vi "RSZVB Set Noise Figure Measurement Mode.vi"(8 "error in (no error)":errorcluster {"code" format="%.0x"}, 9 "Measurement Mode (On)":bool=TRUE, 10 "Channel (1)":i32=1, 11 "VISA session":refnum<visa-resource-name>) -> (0 "error out":errorcluster {"code" format="%.0x"}, 3 "dup VISA session":refnum<visa-resource-name>)   [LabVIEW 2011]
doc: "This VI selects sequential or simultaneous measurement mode. \n\nNote(s):\n\n(1) This VI is available only with option R&S ZVAB-K30.\n\nRemote-control command(s):\n[SENSe<Ch>:]NFIGure:SEQuential ON | OFF"
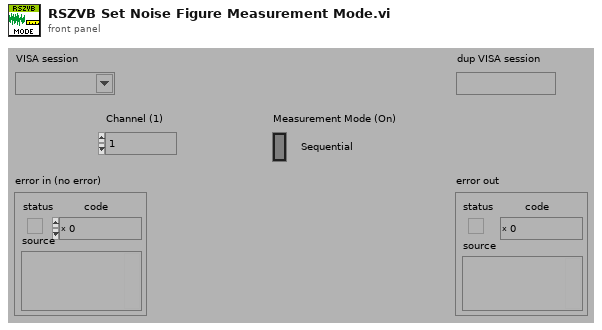
[diagram p1: front panel]
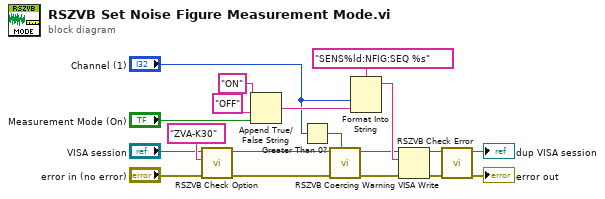
[diagram p0: block diagram]
diagram:
  n1 = call "RSZVB Check Option.vi"("error in (no error)"="error in (no error)", "Options"="ZVA-K30", "VISA session"="VISA session") -> ("error out"=w5:errorcluster, "dup VISA session"=w6:refnum<visa-resource-name>)  [unwired: 7 in]
  n2 = Append True/False String(1:"Measurement Mode (On)", 2:"OFF" ("false string"), 3:"ON" ("true string")) -> (0:w7:string)  [unwired: 1 in]
  n3 = Greater Than 0?(x="Channel (1)") -> (x > 0?=w15:bool)
  n4 = call "RSZVB Coercing Warning.vi"("In Range?"=w15, "error in (no error)"=w5, "VISA session"=w6) -> ("error out"=w14:errorcluster, "dup VISA session"=w13:refnum<visa-resource-name>)  [unwired: 7 in]
  n5 = Format Into String(format string="SENS%ld:NFIG:SEQ %s", "Channel (1)", w7) -> (resulting string=w16:string)  [unwired: 2 in, 1 out]
  n6 = VISA Write(VISA resource name=w13, write buffer=w16, error in (no error)=w14) -> (VISA resource name out=w10:refnum<visa-resource-name>, error out=w11:errorcluster)  [unwired: 1 out]
  n7 = call "RSZVB Check Error.vi"("error in (no error)"=w11, "VISA session"=w10) -> ("error out"=→"error out":errorcluster, "dup VISA session"=→"dup VISA session":refnum<visa-resource-name>)  [unwired: 8 in]
